vi "GetPrivateQueueConfig.vi"(8 "error in (no error)":errorcluster, 11 "Generator":refnum<class "Generator.lvclass">) -> (0 "error out":errorcluster, 3 "Generator out":refnum<class "Generator.lvclass">)   [LabVIEW 2019, in "Generator.lvclass"]
uses:
  Generator.lvclass
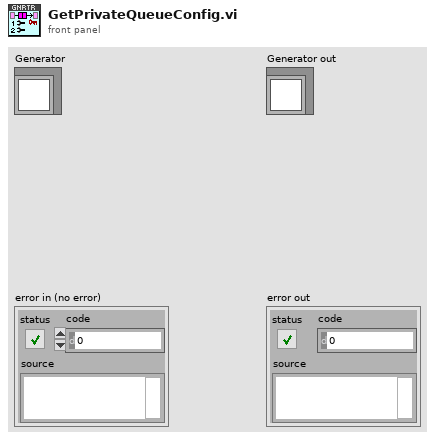
[diagram p1: front panel]
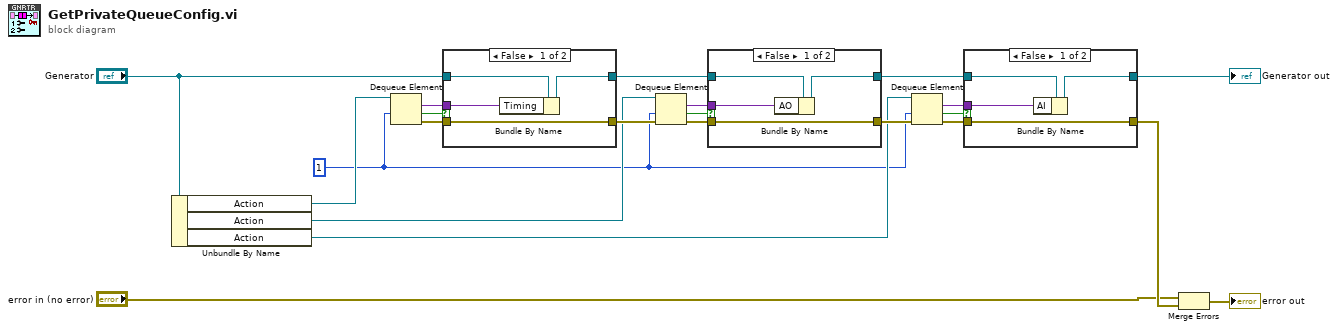
[diagram p0: block diagram]
diagram:
  w1 = 1 ("timeout in ms (-1)")
  n1 = Unbundle By Name("Generator") -> ("Action"=w20:refnum<queue>, "Action"=w8:refnum<queue>, "Action"=w7:refnum<queue>)
  n2 = Dequeue Element(queue=w20, timeout in ms (-1)=w1) -> (element=w19:variant, timed out?=w18:bool, error out=w17:errorcluster)  [unwired: 1 in, 1 out]
  n3 = case shown="False" w18 {
    tunnel: "Generator" -> [w26 w27]
    tunnel: [w25 w27] -> w6
    tunnel: w19 -> [w24 _]
    tunnel: [w23 w28] -> w13
    tunnel: w17 -> [w23 w28]
    frame False {
      n4 = Bundle By Name(cluster=w26, "Timing"=w24) -> (w25:refnum<class "Generator.lvclass">)
    }
    frame True {
    }
  }
  n5 = Dequeue Element(queue=w8, timeout in ms (-1)=w1, error in (no error)=w13) -> (element=w14:variant, timed out?=w15:bool, error out=w16:errorcluster)  [unwired: 1 out]
  n6 = case shown="False" w15 {
    tunnel: w6 -> [w32 w33]
    tunnel: [w31 w33] -> w5
    tunnel: w14 -> [w30 _]
    tunnel: [w29 w34] -> w9
    tunnel: w16 -> [w29 w34]
    frame False {
      n7 = Bundle By Name(cluster=w32, "AO"=w30) -> (w31:refnum<class "Generator.lvclass">)
    }
    frame True {
    }
  }
  n8 = Dequeue Element(queue=w7, timeout in ms (-1)=w1, error in (no error)=w9) -> (element=w12:variant, timed out?=w11:bool, error out=w10:errorcluster)  [unwired: 1 out]
  n9 = case shown="False" w11 {
    tunnel: w5 -> [w38 w39]
    tunnel: [w37 w39] -> w21
    tunnel: w12 -> [w36 _]
    tunnel: [w35 w40] -> w4
    tunnel: w10 -> [w35 w40]
    frame False {
      n10 = Bundle By Name(cluster=w38, "AI"=w36) -> (w37:refnum<class "Generator.lvclass">)
    }
    frame True {
    }
  }
  "Generator out" <- w21
  n11 = Merge Errors("error in (no error)", w4) -> (→"error out":errorcluster)
